vi "create_instance.vi"(8 "error in (no error)":errorcluster, 11 "relative path":string) -> (0 "error out":errorcluster, 3 "FPGAWrapperAN110607Galvo.lvclass":refnum<class "FPGAWrapperAN110607Galvo.lvclass">)   [LabVIEW 2010]
uses:
  FPGAWrapperAN110607Galvo.lvclass
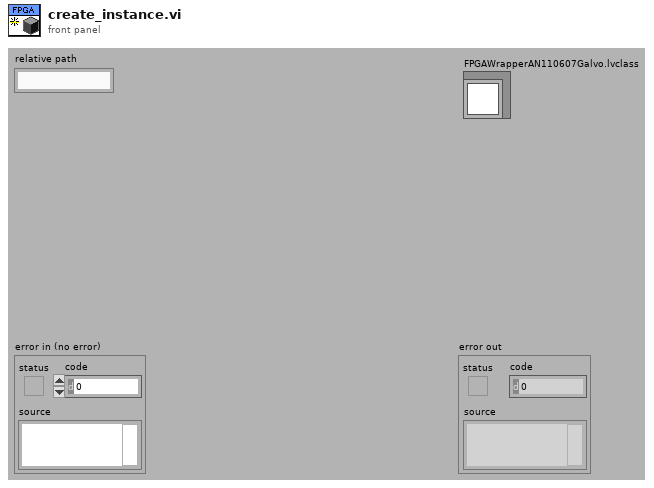
[diagram p1: front panel]
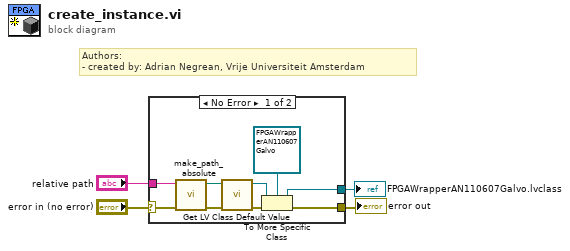
[diagram p0: block diagram]
diagram:
  # "Authors: \n- created by: Adrian Negrean, Vrije Universiteit Amsterdam"
  n1 = case shown="No Error" "error in (no error)" {
    selector: "error in (no error)" -> [w11 w14]
    tunnel: [w10 w14] -> w3
    tunnel: [w6 _] -> w1
    tunnel: "relative path" -> [w9 _]
    frame No Error {
      n2 = call "make_path_absolute.vi"("error in (no error)"=w11, "relative path"=w9) -> ("error out"=w12:errorcluster, "absolute path"=w8:path)  [unwired: 8 in]
      n3 = call <vilib>:"Get LV Class Default Value.vi"("error in (no error)"=w12, "class path"=w8) -> ("error out"=w13:errorcluster, "object"=w7:refnum<class>)  [unwired: 8 out]
      n4 = To More Specific Class(target class=refnum<class "FPGAWrapperAN110607Galvo.lvclass"> refnum ("FPGAWrapperAN110607Galvo.lvclass"), reference=w7, error in=w13) -> (specific class reference=w6:refnum<class "FPGAWrapperAN110607Galvo.lvclass">, error out=w10:errorcluster)
    }
    frame Error {
    }
  }
  "error out" <- w3
  "FPGAWrapperAN110607Galvo.lvclass" <- w1
